vi "Close SQLServer Connection.vi"(8 "error in (no error)":errorcluster, 11 "ADODB._Connection":refnum<k7>) -> (0 "error out":errorcluster)   [LabVIEW 2017]
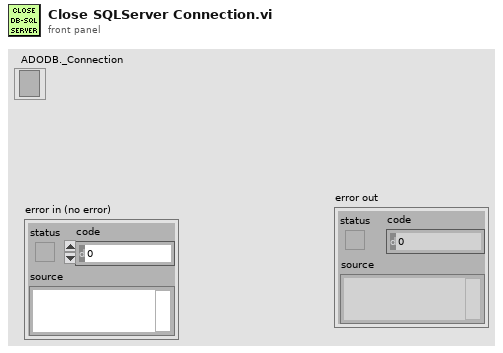
[diagram p1: front panel]
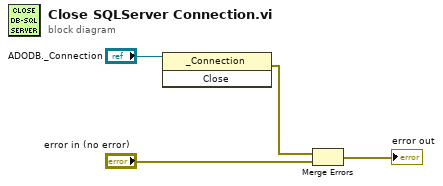
[diagram p0: block diagram]
diagram:
  n1 = invoke class="_Connection" method="Close"(reference="ADODB._Connection") -> (error out=w3:errorcluster)  [unwired: 2 in, 2 out]
  n2 = Merge Errors(w3, "error in (no error)") -> (→"error out":errorcluster)
